vi "GLdrv_AMP_AZERO.vi"(0 "Connection ID":T1, 5 "CH":i32=1 min=1, 7 "AutoZero":enum16{"SET", "RESET"}(ring), 11 "error in (no error)":errorcluster, 13 "Query(f)":bool) -> (4 "Connection ID Out":T1, 10 "Point out":string, 15 "error out":errorcluster)   [LabVIEW 2017, in "GL860_Driver.lvlib"]
doc: "アンプのゼロ点を調節します\nSET：　現在の入力をゼロ点として調節します\nRESet：　ゼロ点調節した設定をリセットします\nPOINT：　ゼロ点調節したオフセットを参照します\n例）:AMP:CH1:AZERO SET (CH1をオートゼロ設定します)\n例）:AMP:CH2:POINT? → :AMP:CH2:POINT 0.12V (CH2のオ\nートゼロオフセット値を参照します)\n※入力信号によってはオートゼロ調節できない場合があります。\n正しくオートゼロが設定できたかはPOINTコマンドを使用してオ\nフセット値を確認してください。"
uses:
  GL860_Driver.lvlib
  ConnectionID.ctl
  GLdrv_RW.ctl
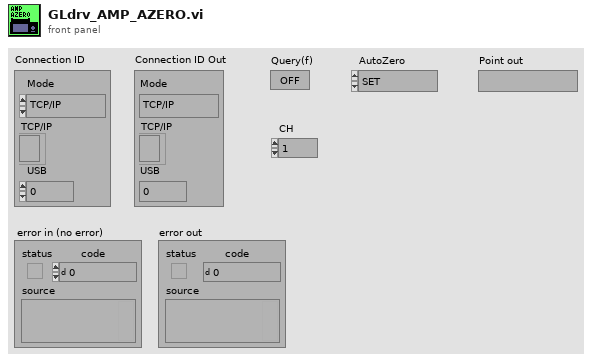
[diagram p1: front panel]
types:
  T1 = typedef "ConnectionID.ctl" = cluster{"Mode":enum16{"TCP/IP", "USB"}, "TCP/IP":refnum<k5>, "USB":i32}
  T2 = typedef "GLdrv_RW.ctl" = enum16{"Auto", "Read", "Write", "Buffer"}
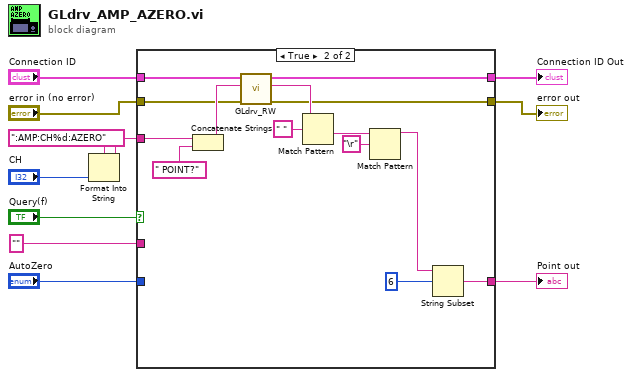
[diagram p0: block diagram]
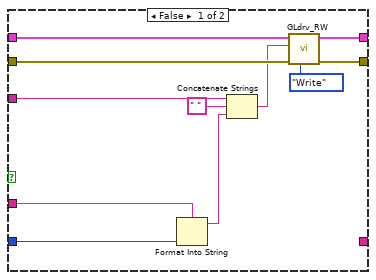
[diagram p2: hidden frame]
diagram:
  n1 = Format Into String(format string=":AMP:CH%d:AZERO" ("Command"), "CH") -> (resulting string=w5:string)  [unwired: 2 in, 1 out]
  n2 = case shown="TRUE" "Query(f)" {
    tunnel: w5 -> [w22 w33]
    tunnel: [w17 w26] -> w11
    tunnel: [w19 w30] -> w10
    tunnel: "Connection ID" -> [w20 w31]
    tunnel: "error in (no error)" -> [w18 w27]
    tunnel: "AutoZero" -> [w13 _]
    tunnel: [_ w25] -> w2
    tunnel: "" ("Param") -> [w12 _]
    frame False {
      n3 = Format Into String(format string=w12, w13) -> (resulting string=w14:string)  [unwired: 2 in, 1 out]
      n4 = Concatenate Strings(w22, " " ("string"), w14) -> (w16:string)
      n5 = call "GLdrv_RW.vi"("Mode(read)"=GLdrv_RW."Write", "error in (no error)"=w18, "data in"=w16, "Connection ID"=w20) -> ("error out"=w17:errorcluster, "Connection ID Out"=w19:T1)  [unwired: 3 in, 3 out]
    }
    frame True {
      n6 = Concatenate Strings(w33, " POINT?" ("string")) -> (w29:string)
      n7 = call "GLdrv_RW.vi"("error in (no error)"=w27, "data in"=w29, "Connection ID"=w31) -> ("error out"=w26:errorcluster, "data out"=w28:string, "Connection ID Out"=w30:T1)  [unwired: 4 in, 2 out]
      n8 = Match Pattern(string=w28, regular expression=" " ("search string/char (-)")) -> (after substring=w34:string)  [unwired: 4 out]
      n9 = Match Pattern(string=w34, regular expression="\r") -> (before substring=w24:string)  [unwired: 4 out]
      n10 = String Subset(string=w24, offset (0)=u32 6 ("initial scan location")) -> (substring=w25:string)  [unwired: 1 out]
    }
  }
  "Connection ID Out" <- w10
  "error out" <- w11
  "Point out" <- w2
